vi "Mój.vi"() -> ()   [LabVIEW 2015]
panel:
  in  "stop":bool
  out "x*y":dbl
  in  "OK Button":bool
  out "Iloœæ wykonania pêtli":i32
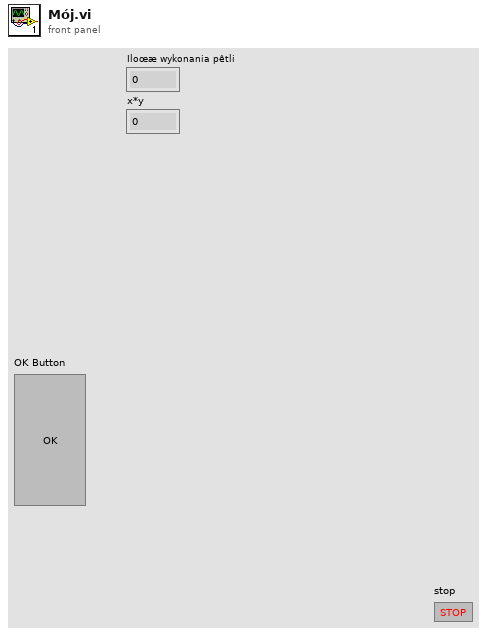
[diagram p1: front panel]
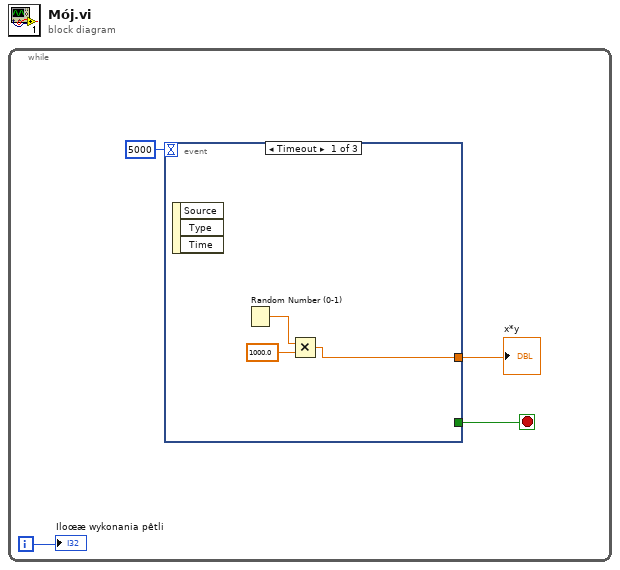
[diagram p0: block diagram]
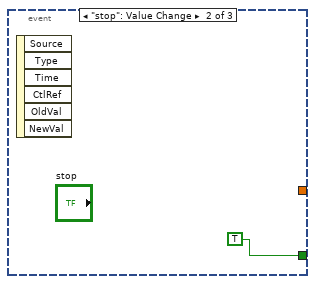
[diagram p2: hidden frame]
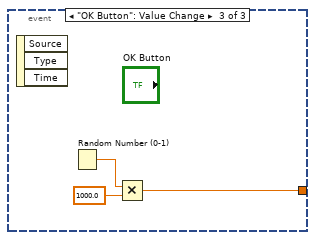
[diagram p3: hidden frame]
diagram:
  n1 = while {
    i -> [w4]
    stop <- w2 stop-if-true
    n2 = event shown="[0] Timeout" {
      selector: _ -> [_ _ _]
      dyn-events: _ -> [_ _ _]
      timeout: 5000 -> [_ _ _]
      tunnel: [w5 _ w9] -> w3
      tunnel: [_ TRUE _] -> w2
      event Timeout {
        n3 = event-data() -> ()  [unwired: 1 in, 3 out]
        n4 = Random Number (0-1)() -> (number: 0 to 1=w6:dbl)
        n5 = Multiply(x=w6, y=1000.0) -> (x*y=w5:dbl)
      }
      event "stop": Value Change {
        n6 = event-data() -> ()  [unwired: 1 in, 6 out]
      }
      event "OK Button": Value Change {
        n7 = event-data() -> ()  [unwired: 1 in, 3 out]
        n8 = Random Number (0-1)() -> (number: 0 to 1=w10:dbl)
        n9 = Multiply(x=w10, y=1000.0) -> (x*y=w9:dbl)
      }
    }
    "x*y" <- w3
    "Iloœæ wykonania pêtli" <- w4
  }
